vi "solar_read VoyagerRefnum.vi"(8 "error in (no error)":errorcluster, 11 "solar in":refnum<class "solar.lvclass">) -> (0 "error out":errorcluster, 2 "VoyagerRefnum":T1, 3 "solar out":refnum<class "solar.lvclass">)   [LabVIEW 2018, in "solar.lvclass"]
doc: "This returns the Voyager refnum which handles communication to COSMOS. Voyager only creates one TCP port by default (this is editable in the configuration files) so that the SOLAR applicaiton appears as one interface in COSMOS."
uses:
  solar.lvclass
  voyager/solar_voy_ctl Voyager Refnum.ctl
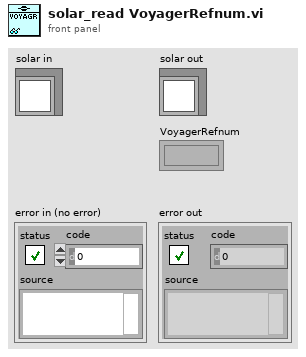
[diagram p1: front panel]
types:
  T1 = typedef "solar_voy_ctl Voyager Refnum.ctl" = refnum<k1>
  T2 = typedef "solar_ctl SOLAR Refnum.ctl" = refnum<k1>
  T3 = typedef "solar_ctl SOLAR Global.ctl" = cluster{"Targets":T4[], "AppDir":path, "solar.ini":path, "ConfigsDir":path, "CosmosDir":path, "LogsDir":path, "ExePath":path, "ExeVersion":string, "PartNum":string, "AppSetup":string, "Title":string, "Main.ini":path, "Temp.ini":path, "vSOLAR":string, "Splash.png":string, "SplashWait":i32, "SOLARUE":refnum<user-event>, "VoyagerRefnum":T1, "QTimerRefnum":T5}
  T4 = typedef "solar_ctl Target Global.ctl" = cluster{"Target":string, "Q":refnum<queue>, "UE":refnum<user-event>, "VI":refnum<vi>, "Menu":refnum<k9>, "Data":refnum<data-value>, "Attributes":variant}
  T5 = typedef "solar_qtimer_ctl Refnum.ctl" = refnum<k1>
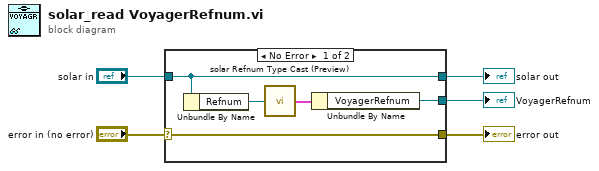
[diagram p0: block diagram]
diagram:
  n1 = case shown="No Error" "error in (no error)" {
    selector: "error in (no error)" -> [w7 w12]
    tunnel: "solar in" -> [w6 w11]
    tunnel: [w8 _] -> w4
    tunnel: [w7 w12] -> w3
    tunnel: [w6 w11] -> w1
    frame No Error {
      n2 = Unbundle By Name(w6) -> ("Refnum"=w10:T2)
      n3 = call "solar Refnum Type Cast (Preview).vi"("Refnum"=w10) -> ("SOLAR"=w9:T3)  [unwired: 8 in]
      n4 = Unbundle By Name(w9) -> ("VoyagerRefnum"=w8:T1)
    }
    frame Error {
    }
  }
  "error out" <- w3
  "solar out" <- w1
  "VoyagerRefnum" <- w4
